vi "Update SubPanel Size.vi"(8 "error in (no error)":errorcluster, 10 "Window Size":T1, 11 "SubPanel in":refnum<vi>) -> (0 "error out":errorcluster)   [LabVIEW 2020, in "Group Interface.lvlib"]
uses:
  <vilib>/Utility/miscctls.llb/LVRectTypeDef.ctl
  <vilib>/Utility/miscctls.llb/LVBoundsTypeDef.ctl
  Group Interface.lvlib
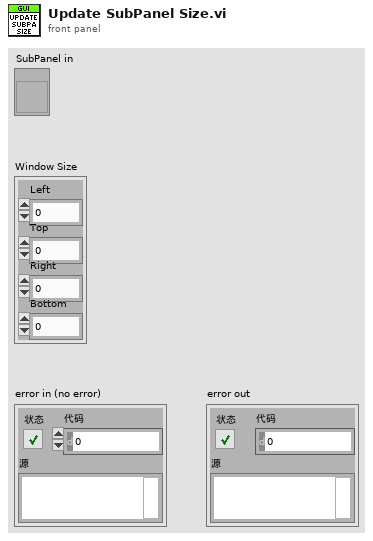
[diagram p1: front panel]
types:
  T1 = typedef "LVRectTypeDef.ctl" = cluster{"Left":i16, "Top":i16, "Right":i16, "Bottom":i16}
  T2 = typedef "LVBoundsTypeDef.ctl" = cluster{"Width":u32, "Height":u32}
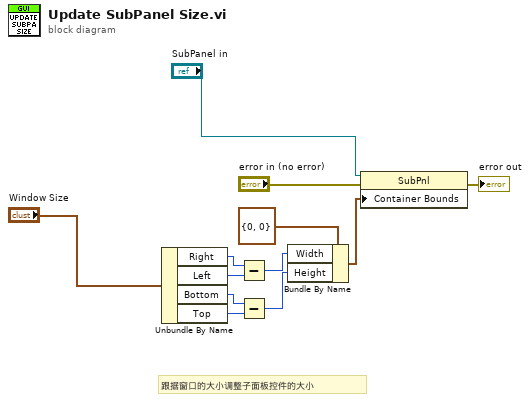
[diagram p0: block diagram]
diagram:
  # "跟据窗口的大小调整子面板控件的大小"
  n1 = Unbundle By Name("Window Size") -> ("Right"=w6:i16, "Left"=w5:i16, "Bottom"=w3:i16, "Top"=w2:i16)
  n2 = Subtract(x=w6, y=w5) -> (x-y=w4:i16)
  n3 = Subtract(x=w3, y=w2) -> (x-y=w1:i16)
  n4 = Bundle By Name(cluster=T2 {"Width"=0, "Height"=0} ("容器边界"), "Width"=w4, "Height"=w1) -> (w7:T2)
  n5 = property class="SubPnl"(reference="SubPanel in", error in="error in (no error)", "Container Bounds"=w7) -> (error out=→"error out":errorcluster)  [unwired: 1 out]
